vi "Import SLSC Switch Custom Device.vi"(8 "error in":errorcluster, 10 "datalog path (use dialog)":path, 11 "slsc switch custom device in":T1 format="%.0x") -> (0 "error out":errorcluster, 3 "slsc switch custom device out":T1 format="%.0x")   [LabVIEW 2017, in "NI-SWITCH Scripting.lvlib"]
doc: "Replaces the existing SLSC Switch custom device configuration with the configuration specified by a datalog file. Create the datalog file by using <b>Export SLSC Switch Custom Device.vi</b>."
uses:
  NI-SWITCH Scripting.lvlib
  <vilib>/NI Veristand/Custom Device API/Custom Device Item Ref.ctl
  <vilib>/NI Veristand/Custom Device API/Get Item Property (I32).vi
  <vilib>/NI Veristand/Custom Device API/Set Item Property (I32).vi
  <vilib>/NI/NI VeriStand Custom Device Import and Export Tool/ImportExport.lvlib
  <vilib>/NI VeriStand/Custom Device API/Custom Device API.lvlib
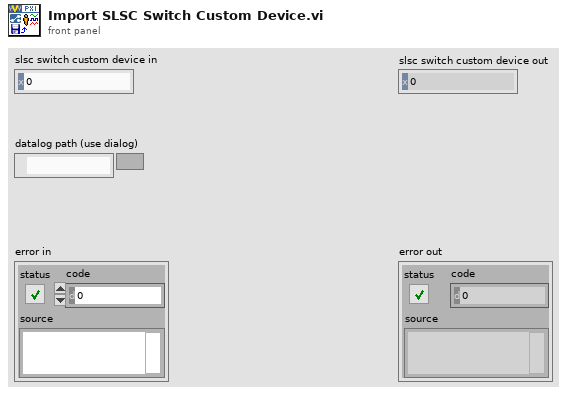
[diagram p1: front panel]
types:
  T1 = typedef "Custom Device API.lvlib/Custom Device Item Ref.ctl" = u64
  T2 = typedef "NI-SWITCH Shared.lvlib/Endpoint Configuration Cluster.ctl" = cluster{"Endpoint":string, "Configuration":T3}
  T3 = typedef "NI-SWITCH Shared.lvlib/Endpoint Configuration Enum.ctl" = enum16{"Load", "Source", "Configuration"}
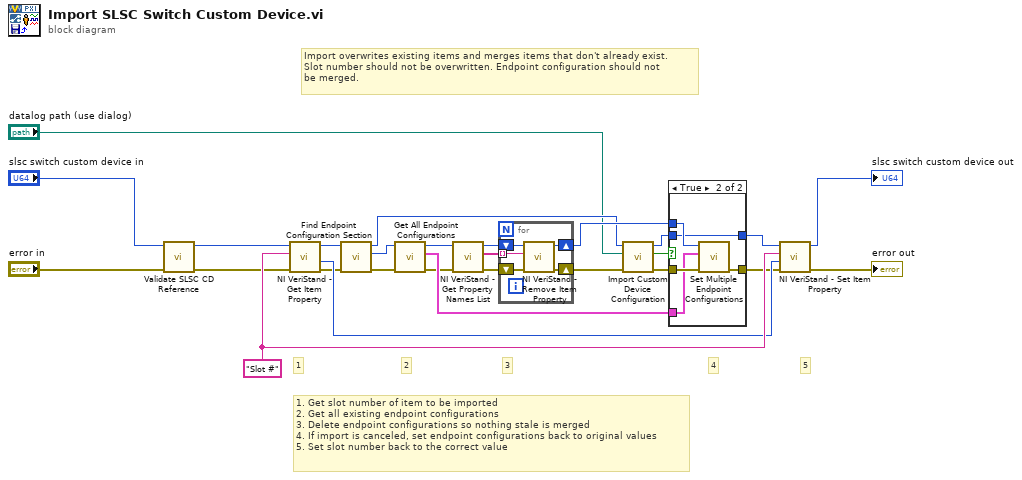
[diagram p0: block diagram]
diagram:
  w27 = "Slot #" ("Property Name")
  # "1. Get slot number of item to be imported\n2. Get all existing endpoint configurations\n3. Delete endpoint configurations so nothing stale is merged\n4. If import is canceled, set endpoint configurations back to original values\n5. Set slot number back to the correct value"
  # "5"
  # "4"
  # "3"
  # "2"
  # "1"
  # "Import overwrites existing items and merges items that don't already exist.\nSlot number should not be overwritten. Endpoint configuration should not\nbe merged."
  n1 = call "Validate SLSC CD Reference.vi"("error in"="error in", "slsc switch custom device in"="slsc switch custom device in") -> ("error out"=w3:errorcluster, "slsc switch custom device out"=w1:T1)  [unwired: 8 in]
  n2 = call-poly <vilib>:"NI VeriStand - Get Item Property.vi"("error in (no error)"=w3, "Property Name"=w27, "Item Ref in"=w1) -> ("error out"=w19:errorcluster, "Value"=w26:i32, "Item Ref out"=w18:T1)  [unwired: 5 in, 1 out]
  n3 = call "Find Endpoint Configuration Section.vi"("error in"=w19, "slsc switch custom device in"=w18) -> ("error out"=w16:errorcluster, "endpoint configuration"=w17:T1, "slsc switch custom device out"=w8:T1)  [unwired: 7 in]
  n4 = call "Get All Endpoint Configurations.vi"("error in"=w16, "endpoint configuration in"=w17) -> ("error out"=w15:errorcluster, "endpoint configurations"=w20:T2[], "endpoint configuration out"=w13:T1)  [unwired: 7 in]
  n5 = call <vilib>:"NI VeriStand - Get Property Names List.vi"("error in (no error)"=w15, "Item Ref in"=w13) -> ("error out"=w14:errorcluster, "Property Names"=w11:string[], "Item Ref out"=w12:T1)  [unwired: 7 in]
  n6 = for {
    shift-right: [w30] -> w9
    shift-left: w14 -> [w32]
    shift-right: [w29] -> w10
    shift-left: w12 -> [w31]
    tunnel: w11 -> [w28] mode=indexing
    n7 = call <vilib>:"NI VeriStand - Remove Item Property.vi"("error in (no error)"=w32, "Property Name"=w28, "Item Ref in"=w31) -> ("error out"=w30:errorcluster, "Item Ref out"=w29:T1)  [unwired: 6 in, 1 out]
  }
  n8 = call <vilib>:"Import Custom Device Configuration.vi"("error in (no error)"=w9, "Path"="datalog path (use dialog)", "NodeID"=w8) -> ("error out"=w25:errorcluster, "cancelled"=w22:bool, "NodeID out"=w21:u64)  [unwired: 6 in]
  n9 = case shown="True" w22 {
    tunnel: w25 -> [w34 w39]
    tunnel: [w34 w38] -> w24
    tunnel: [w33 w35] -> w23
    tunnel: w21 -> [w33 w35]
    tunnel: w20 -> [_ w37]
    tunnel: w10 -> [_ w36]
    frame False {
    }
    frame True {
      n10 = call "Set Multiple Endpoint Configurations.vi"("error in"=w39, "endpoint configurations"=w37, "endpoint configuration in"=w36) -> ("error out"=w38:errorcluster)  [unwired: 7 in, 1 out]
    }
  }
  n11 = call-poly <vilib>:"NI VeriStand - Set Item Property.vi"("error in (no error)"=w24, "Value"=w26, "Property Name"=w27, "Item Ref in"=w23) -> ("error out"=→"error out":errorcluster, "Item Ref out"=→"slsc switch custom device out":T1)  [unwired: 5 in, 1 out]
